vi "testMatrix_load_DELAY_fpga.vi"() -> ()   [LabVIEW 2017]
uses:
  <vilib>/rvi/DataTransferAndStorage/Container/Common/niFpgaContainerExecOnDevCompGetState.vi
  <vilib>/rvi/Emulation/niFpgaEmulationIsFPGAContextNoSignature.vi
  <vilib>/rvi/DataTransferAndStorage/Container/Common/niFpgaContainerGetUniqueNameForEmu.vi
  <vilib>/rvi/Emulation/niFpgaProcessEmulError.vi
  <vilib>/rvi/Emulation/niFpgaSctlEmulationGetInTimedLoop.vi
  <vilib>/rvi/errors/nirviReportUnexpectedCaseInternalError (U32).vi
  <vilib>/rvi/Memory/Memory_Emulation/niFpgaMemoryEmulationCacheClearOnFirstRun.vi
  <vilib>/rvi/Memory/Memory_Emulation/nirvimemoryEmulationManagerCache_MakeExclusive.vi
  <vilib>/rvi/Memory/Memory_Emulation/niFpgaMemoryEmulationValidateCache.vi
  <vilib>/rvi/Memory/Memory_Emulation/nirvimemoryEmulationManagerCache_InsertValue.vi
  <vilib>/Utility/error.llb/Clear Errors.vi
  <vilib>/rvi/Memory/Memory_Emulation/nirvimemoryEmulationManagerCache_ReleaseExclusive.vi
  <vilib>/rvi/Memory/Memory_Emulation/nirvimemoryEmulationManagerCache_GetValue.vi
  <vilib>/rvi/Memory/Memory_Emulation/nirvimemoryEmulationManagerCache_SetValue.vi
  <vilib>/rvi/Emulation/niFpgaSctlEmulationResourceMgr.vi
  <vilib>/rvi/DataTransferAndStorage/Container/XNode/niFpgaContainer.xnode
  <vilib>/rvi/Memory/Memory_Emulation/niFpgaMemoryEmulationRefIn.vi
panel:
  out "C":sgl[](array[numeric])=[0.0022478297, 0.0, 0.0, 0.0, 0.0, 0.0, 0.0, 0.0, 0.0, 0.0, 0.0, 0.0]
  out "Kdelay":sgl[](array[numeric])=[0.0022478297, 0.0, 0.0, 0.0, 0.0, 0.0, 0.0, 0.0, 0.0, 0.0, 0.0, 0.0]
  out "K":sgl[](array[numeric])=[0.0022478297, 0.0, 0.0, 0.0, 0.0, 0.0, 0.0, 0.0, 0.0, 0.0, 0.0, 0.0]
  in  "ND":i16
  out "Aascol":sgl[](array[numeric])=[0.0022478297, 0.0, 0.0, 0.0, 0.0, 0.0, 0.0, 0.0, 0.0, 0.0, 0.0, 0.0, 0.0, 0.0, 0.0, 0.0, 0.0, 0.0, 0.0, 0.0, 0.0, 0.0, 0.0, 0.0, 0.0, 0.0, 0.0, 0.0, 0.0, 0.0, 0.0, 0.0, 0.0, 0.0, 0.0, 0.0, 0.0, 0.0, 0.0, 0.0, 0.0, 0.0, 0.0, 0.0, 0.0, 0.0, 0.0, 0.0, 0.0, 0.0, 0.0, 0.0, 0.0, 0.0, 0.0, 0.0, 0.0, 0.0, 0.0, 0.0, 0.0, 0.0, 0.0, 0.0, 0.0, 0.0, 0.0, 0.0, 0.0, 0.0, 0.0, 0.0, 0.0, 0.0, 0.0, 0.0, 0.0, 0.0, 0.0, 0.0, 0.0, 0.0, 0.0, 0.0, 0.0, 0.0, 0.0, 0.0, 0.0, 0.0, 0.0, 0.0, 0.0, 0.0, 0.0, 0.0, 0.0, 0.0, 0.0, 0.0, 0.0, 0.0, 0.0, 0.0, 0.0, 0.0, 0.0, 0.0, 0.0, 0.0, 0.0, 0.0, 0.0, 0.0, 0.0, 0.0, 0.0, 0.0, 0.0, 0.0, 0.0, 0.0, 0.0, 0.0, 0.0, 0.0, 0.0, 0.0, 0.0, 0.0, 0.0, 0.0, 0.0, 0.0, 0.0, 0.0, 0.0, 0.0, 0.0, 0.0, 0.0, 0.0, 0.0, 0.0]
  out "Bz":sgl[](array[numeric])=[0.0022478297, 0.0, 0.0, 0.0, 0.0, 0.0, 0.0, 0.0, 0.0, 0.0, 0.0, 0.0]
  out "L":sgl[](array[numeric])=[0.0022478297, 0.0, 0.0, 0.0, 0.0, 0.0, 0.0, 0.0, 0.0, 0.0, 0.0, 0.0]
  in  "NS":i16
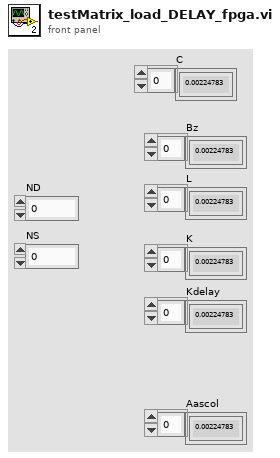
[diagram p1: front panel]
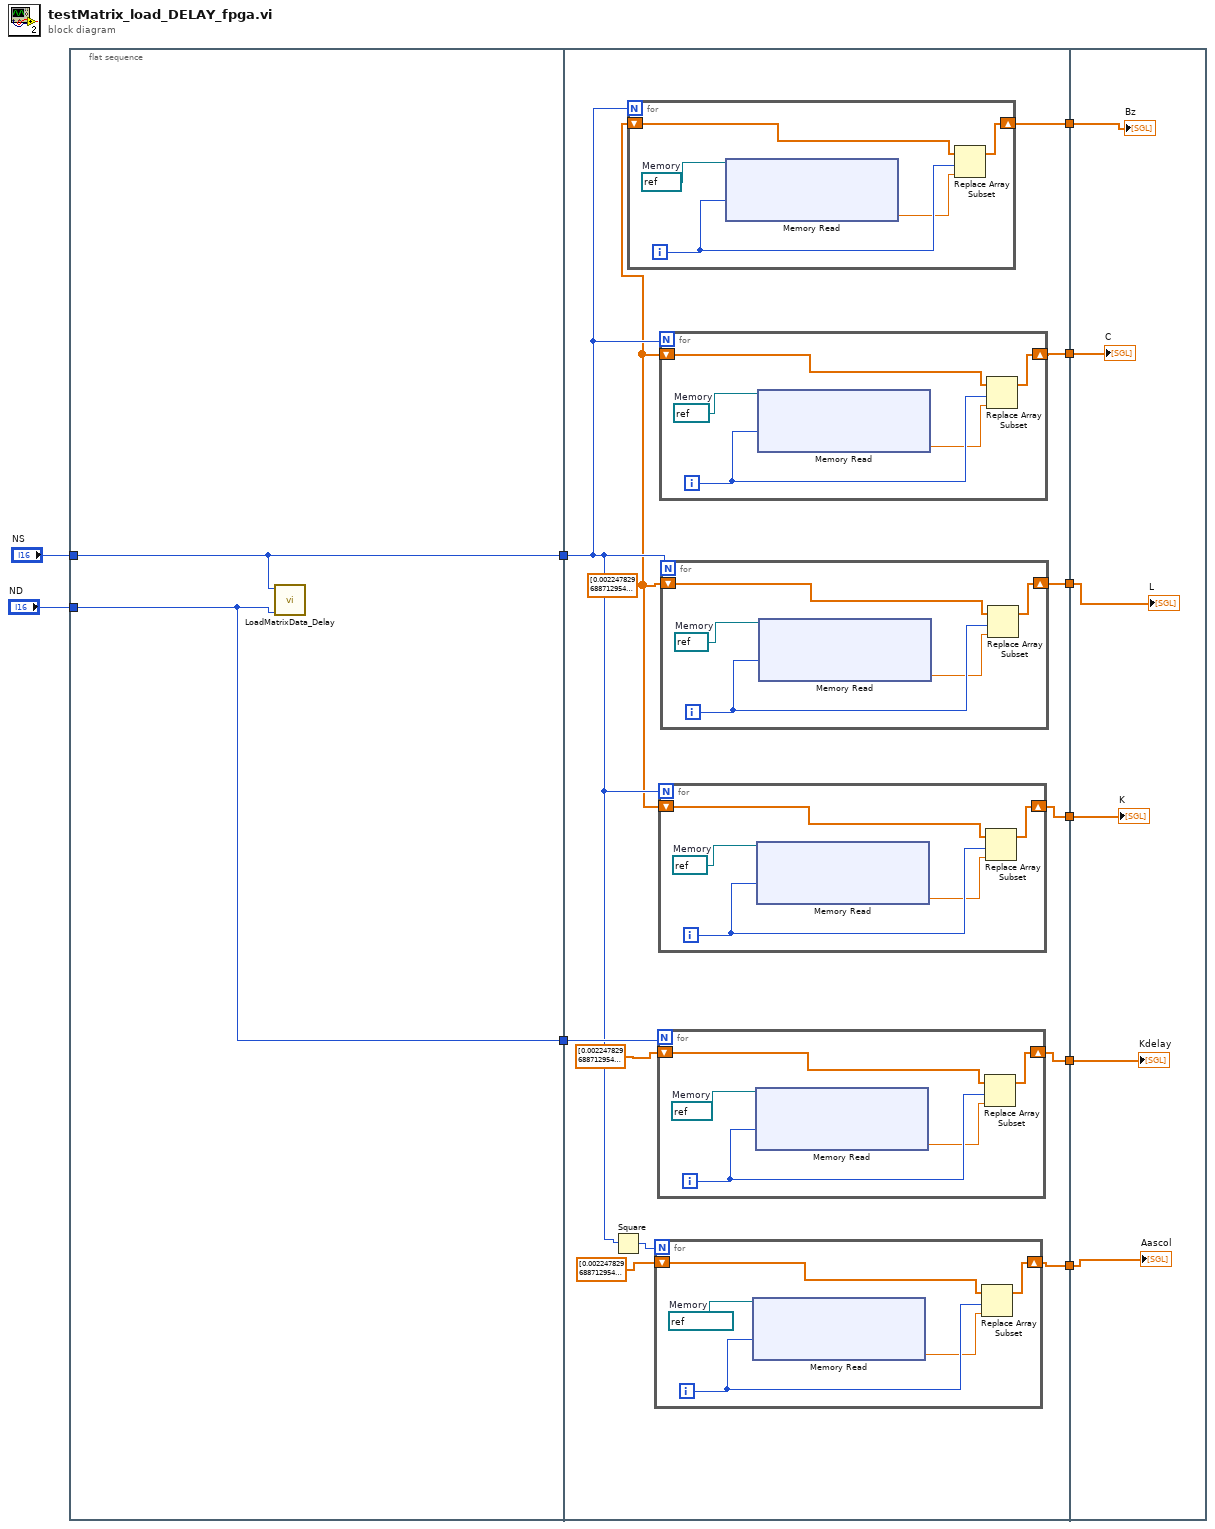
[diagram p0: block diagram]
diagram:
  n1 = flat-sequence {
    tunnel: "NS" -> [w12]
    tunnel: [w12] -> w8
    tunnel: "ND" -> [w11]
    tunnel: [w11] -> w3
    tunnel: [w24] -> w9
    tunnel: w8 -> [w15]
    tunnel: [w23] -> w7
    tunnel: [w22] -> w6
    tunnel: [w21] -> w5
    tunnel: w3 -> [w20]
    tunnel: [w18] -> w2
    tunnel: [w13] -> w1
    tunnel: w9 -> [w60]
    tunnel: w7 -> [w59]
    tunnel: w6 -> [w57]
    tunnel: w5 -> [w58]
    tunnel: w2 -> [w56]
    tunnel: w1 -> [w55]
    frame #0 {
      n2 = call "LoadMatrixData_Delay.vi"("Nd"=w11, "NS"=w12) -> ()  [unwired: 9 in, 1 out]
    }
    frame #1 {
      w14 = sgl[] [0.0022478297, 0.0, 0.0, 0.0, 0.0, 0.0, 0.0, 0.0, 0.0, 0.0, 0.0, 0.0] ("All matrix")
      n3 = Square(x=w15) -> (x^2=w17:i16)
      n4 = for {
        N: w15 -> [_]
        shift-right: [w49] -> w23
        shift-left: w14 -> [w48]
        i -> [w46]
        w47 = refnum<k21> "Bz"  # Memory
        n5 = xnode ("Memory Read")("Address"=w46, "Memory In"=w47) -> ("Data"=w45:sgl)  [unwired: 1 out]
        n6 = Replace Array Subset(array=w48, new element=w45, index=w46) -> (w49:sgl[])
      }
      n7 = for {
        N: w17 -> [_]
        shift-right: [w39] -> w21
        shift-left: sgl[] [0.0022478297, 0.0, 0.0, 0.0, 0.0, 0.0, 0.0, 0.0, 0.0, 0.0, 0.0, 0.0, 0.0, 0.0, 0.0, 0.0, 0.0, 0.0, 0.0, 0.0, 0.0, 0.0, 0.0, 0.0, 0.0, 0.0, 0.0, 0.0, 0.0, 0.0, 0.0, 0.0, 0.0, 0.0, 0.0, 0.0, 0.0, 0.0, 0.0, 0.0, 0.0, 0.0, 0.0, 0.0, 0.0, 0.0, 0.0, 0.0, 0.0, 0.0, 0.0, 0.0, 0.0, 0.0, 0.0, 0.0, 0.0, 0.0, 0.0, 0.0, 0.0, 0.0, 0.0, 0.0, 0.0, 0.0, 0.0, 0.0, 0.0, 0.0, 0.0, 0.0, 0.0, 0.0, 0.0, 0.0, 0.0, 0.0, 0.0, 0.0, 0.0, 0.0, 0.0, 0.0, 0.0, 0.0, 0.0, 0.0, 0.0, 0.0, 0.0, 0.0, 0.0, 0.0, 0.0, 0.0, 0.0, 0.0, 0.0, 0.0, 0.0, 0.0, 0.0, 0.0, 0.0, 0.0, 0.0, 0.0, 0.0, 0.0, 0.0, 0.0, 0.0, 0.0, 0.0, 0.0, 0.0, 0.0, 0.0, 0.0, 0.0, 0.0, 0.0, 0.0, 0.0, 0.0, 0.0, 0.0, 0.0, 0.0, 0.0, 0.0, 0.0, 0.0, 0.0, 0.0, 0.0, 0.0, 0.0, 0.0, 0.0, 0.0, 0.0, 0.0] ("All matrix") -> [w38]
        i -> [w36]
        w37 = refnum<k21> "AasCol"  # Memory
        n8 = xnode ("Memory Read")("Address"=w36, "Memory In"=w37) -> ("Data"=w35:sgl)  [unwired: 1 out]
        n9 = Replace Array Subset(array=w38, new element=w35, index=w36) -> (w39:sgl[])
      }
      n10 = for {
        N: w20 -> [_]
        shift-right: [w44] -> w22
        shift-left: sgl[] [0.0022478297, 0.0, 0.0, 0.0, 0.0, 0.0, 0.0, 0.0, 0.0, 0.0, 0.0, 0.0] ("All matrix") -> [w43]
        i -> [w41]
        w42 = refnum<k21> "K2"  # Memory
        n11 = xnode ("Memory Read")("Address"=w41, "Memory In"=w42) -> ("Data"=w40:sgl)  [unwired: 1 out]
        n12 = Replace Array Subset(array=w43, new element=w40, index=w41) -> (w44:sgl[])
      }
      n13 = for {
        N: w15 -> [_]
        shift-right: [w34] -> w18
        shift-left: w14 -> [w33]
        i -> [w31]
        w32 = refnum<k21> "K"  # Memory
        n14 = xnode ("Memory Read")("Address"=w31, "Memory In"=w32) -> ("Data"=w30:sgl)  [unwired: 1 out]
        n15 = Replace Array Subset(array=w33, new element=w30, index=w31) -> (w34:sgl[])
      }
      n16 = for {
        N: w15 -> [_]
        shift-right: [w29] -> w13
        shift-left: w14 -> [w28]
        i -> [w26]
        w27 = refnum<k21> "C"  # Memory
        n17 = xnode ("Memory Read")("Address"=w26, "Memory In"=w27) -> ("Data"=w25:sgl)  [unwired: 1 out]
        n18 = Replace Array Subset(array=w28, new element=w25, index=w26) -> (w29:sgl[])
      }
      n19 = for {
        N: w15 -> [_]
        shift-right: [w54] -> w24
        shift-left: w14 -> [w53]
        i -> [w51]
        w52 = refnum<k21> "L"  # Memory
        n20 = xnode ("Memory Read")("Address"=w51, "Memory In"=w52) -> ("Data"=w50:sgl)  [unwired: 1 out]
        n21 = Replace Array Subset(array=w53, new element=w50, index=w51) -> (w54:sgl[])
      }
    }
    frame #2 {
      "L" <- w60
      "Bz" <- w59
      "Aascol" <- w58
      "K" <- w56
      "Kdelay" <- w57
      "C" <- w55
    }
  }
